vi "CreateQueueNames.vi"(8 "error in (no error)":errorcluster, 11 "ModuleAdmin In":refnum<class "ModuleAdmin.lvclass">) -> (0 "error out":errorcluster, 1 "Class Queue Name":string, 2 "QMH Queue Name":string, 3 "ModuleAdmin Out":refnum<class "ModuleAdmin.lvclass">, 4 "SP Loop Queue Name":string)   [LabVIEW 2018, in "SensorPlugins.lvlib"]
doc: "This VI creates three queue names for the sensor plugin to use based upon a unique module ID."
uses:
  SensorPlugins.lvlib
  <userlib>/NIST/ModuleAdminLib/ModuleAdmin/ModuleAdmin.lvclass
panel:
  in  "QueueNames":string[](array[string])=["QMH", "Class", "SP"]
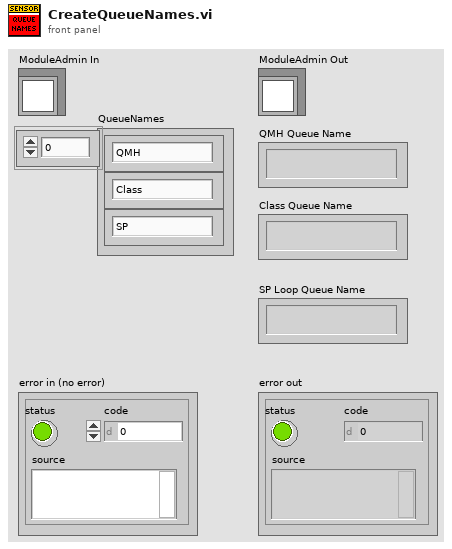
[diagram p1: front panel]
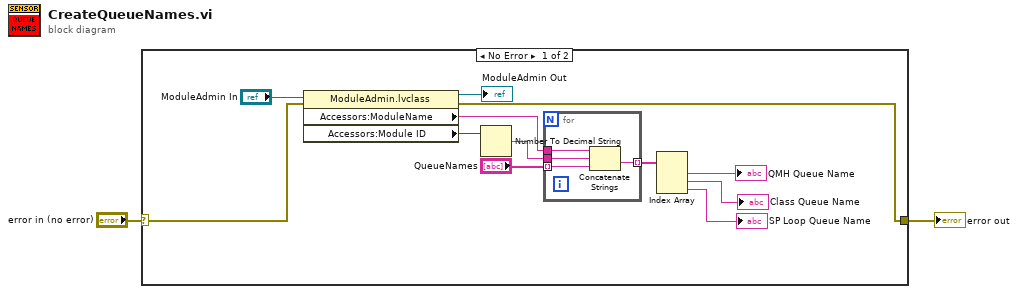
[diagram p0: block diagram]
diagram:
  n1 = case shown="No Error" "error in (no error)" {
    selector: "error in (no error)" -> [w8 w19]
    tunnel: [w7 w19] -> w2
    frame No Error {
      n2 = property class="ModuleAdmin.lvclass"(reference="ModuleAdmin In", error in=w8) -> (reference out=→"ModuleAdmin Out":refnum<class "ModuleAdmin.lvclass">, error out=w7:errorcluster, "Accessors:ModuleName"=w3:string, "Accessors:Module ID"=w4:i32)
      n3 = Number To Decimal String(number=w4) -> (decimal integer string=w5:string)  [unwired: 1 in]
      n4 = for {
        tunnel: [w18] -> w14 mode=indexing
        tunnel: w5 -> [w17]
        tunnel: "QueueNames" -> [w16] mode=indexing
        tunnel: w3 -> [w15]
        n5 = Concatenate Strings(w15, w17, w16) -> (w18:string)
      }
      n6 = Index Array(array=w14) -> (element #1=→"QMH Queue Name":string, element #2=→"Class Queue Name":string, element #3=→"SP Loop Queue Name":string)  [unwired: 3 in]
    }
    frame Error {
    }
  }
  "error out" <- w2
